vi "Unflatten.vi"(8 "error in (no error)":errorcluster, 10 "Buffer":u8[](array[numeric]) format="%.0x", 11 "Msg in":refnum<class "Msg.lvclass">) -> (0 "error out":errorcluster, 3 "Msg out":refnum<class "Msg.lvclass">)   [LabVIEW 2020, in "Error.lvlib" / "Msg.lvclass"]
uses:
  Msg.lvclass
  Msg.lvclass/Msg.ctl
  Error.lvlib
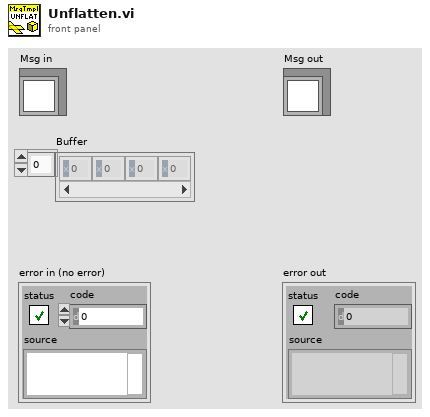
[diagram p1: front panel]
types:
  T1 = typedef "Error.lvlib/Data.ctl" = cluster{"Scalar":dbl, "Array":dbl[]}
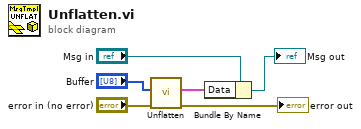
[diagram p0: block diagram]
diagram:
  n1 = call "Unflatten.vi"("error in"="error in (no error)", "Buffer"="Buffer") -> ("error out"=→"error out":errorcluster, "Data"=w2:T1)  [unwired: 8 in]
  n2 = Bundle By Name(cluster="Msg in", "Data"=w2) -> (→"Msg out":refnum<class "Msg.lvclass">)
